vi "15.Evd.5_Ask.5.vi"() -> ()   [LabVIEW 2025]
panel:
  out "1":bool
  out "2":bool
  out "3":bool
  out "4":bool
  out "5 - DANGER":bool
  out "Message":string
  in  "stop":bool
  in  "Engine Speed":dbl(slide) scale=0.0..5.0
  out "RPM":dbl(knob) scale=0.0..50000.0
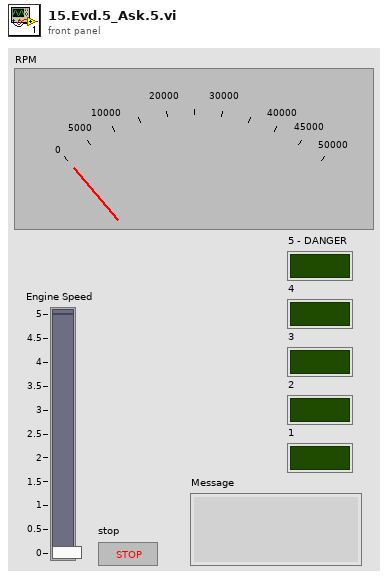
[diagram p1: front panel]
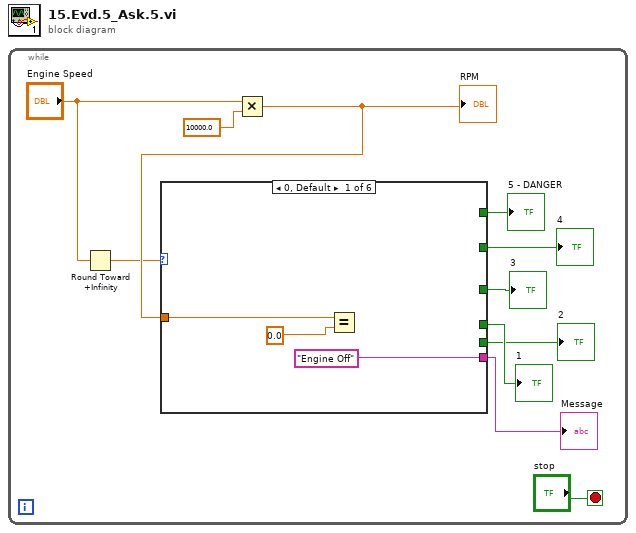
[diagram p0: block diagram]
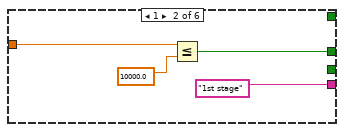
[diagram p2: hidden frame]
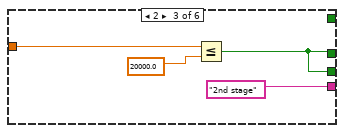
[diagram p3: hidden frame]
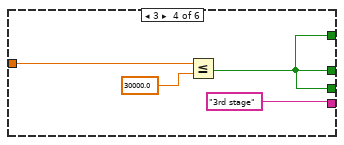
[diagram p4: hidden frame]
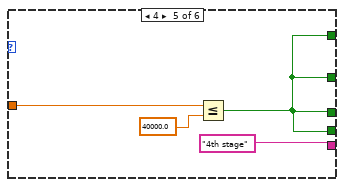
[diagram p5: hidden frame]
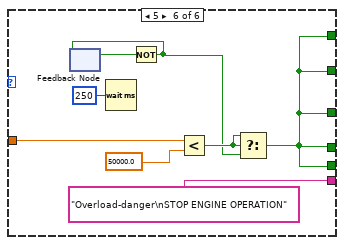
[diagram p6: hidden frame]
diagram:
  n1 = while {
    stop <- "stop" stop-if-true
    n2 = Round Toward +Infinity(x="Engine Speed") -> (ceil(x): smallest int >= x=w2:dbl)
    n3 = Multiply(x="Engine Speed", y=10000.0) -> (x*y=w10:dbl)
    "RPM" <- w10
    n4 = case shown="0, Default" w2 {
      tunnel: w10 -> [w13 w18 w21 w26 w29 w34]
      tunnel: ["Engine Off" "1st stage" "2nd stage" "3rd stage" "4th stage" "Overload-danger\nSTOP ENGINE OPERATION"] -> w1
      tunnel: [_ w15 w19 w23 w28 w32] -> w9
      tunnel: [_ _ w19 w23 w28 w32] -> w8
      tunnel: [_ _ _ w23 w28 w32] -> w7
      tunnel: [_ _ _ _ w28 w32] -> w6
      tunnel: [_ _ _ _ _ w32] -> w5
      frame 0, Default {
        n5 = Equal?(x=w13, y=0.0) -> ()  [unwired: 1 out]
      }
      frame 1 {
        n6 = Less Or Equal?(x=w18, y=10000.0) -> (x <= y?=w15:bool)
      }
      frame 2 {
        n7 = Less Or Equal?(x=w21, y=20000.0) -> (x <= y?=w19:bool)
      }
      frame 3 {
        n8 = Less Or Equal?(x=w26, y=30000.0) -> (x <= y?=w23:bool)
      }
      frame 4 {
        n9 = Less Or Equal?(x=w29, y=40000.0) -> (x <= y?=w28:bool)
      }
      frame 5 {
        n10 = feedback #1() -> (w36:bool)  [unwired: 1 in]
        n11 = Wait (ms)(milliseconds to wait=u32 250) -> ()  [unwired: 1 out]
        n12 = Not(x=w36) -> (.not. x?=w31:bool)
        n13 = feedback-in #1(w31) -> ()
        n14 = Less?(x=w34, y=50000.0) -> (x < y?=w33:bool)
        n15 = Select(t=w33, s=w33, f=w31) -> (s? t:f=w32:bool)
      }
    }
    "Message" <- w1
    "5 - DANGER" <- w5
    "4" <- w6
    "3" <- w7
    "2" <- w8
    "1" <- w9
  }
